vi "Write configuration.vi"(8 "error in":errorcluster, 10 "configuration":refnum<class "NISE_CEF_serializable configuration.lvclass">, 11 "CVT Engine Editor in":refnum<class "CVT Engine Editor.lvclass">) -> (0 "error out":errorcluster, 3 "CVT Engine Editor out":refnum<class "CVT Engine Editor.lvclass">)   [LabVIEW 2013, in "CVT Engine Editor.lvclass"]
uses:
  CVT Engine Editor.lvclass
  <vilib>/NI/Configuration Framework/serializable configuration/NISE_CEF_serializable configuration.lvclass
  Configuration/CVT Engine Configuration.lvclass
  CVT Engine Editor.lvclass/CVT Engine Editor.ctl
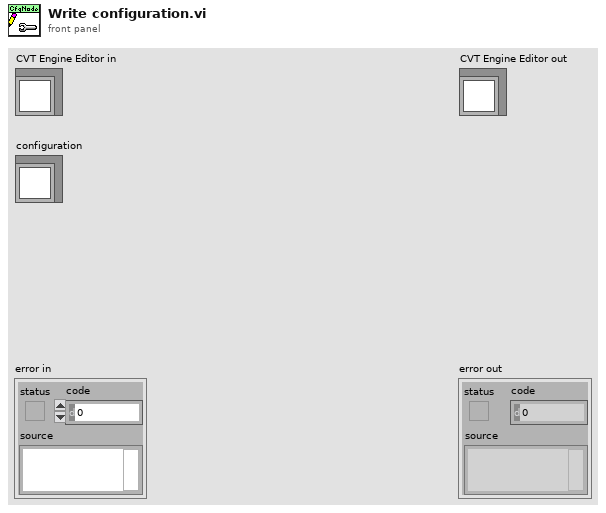
[diagram p1: front panel]
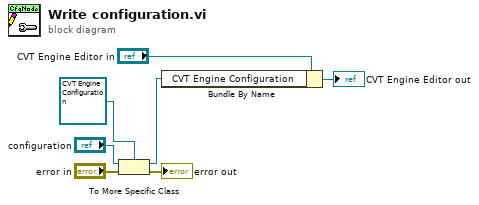
[diagram p0: block diagram]
diagram:
  n1 = To More Specific Class(target class=refnum<class "CVT Engine Configuration.lvclass"> refnum ("CVT Engine Configuration"), reference="configuration", error in="error in") -> (specific class reference=w2:refnum<class "CVT Engine Configuration.lvclass">, error out=→"error out":errorcluster)
  n2 = Bundle By Name(cluster="CVT Engine Editor in", "CVT Engine Configuration"=w2) -> (→"CVT Engine Editor out":refnum<class "CVT Engine Editor.lvclass">)
